vi "Check FET Test.vi"() -> ()   [LabVIEW 2009]
panel:
  in  "STOP":bool
  in  "Check FET":bool
  out "FETs on?":bool=TRUE
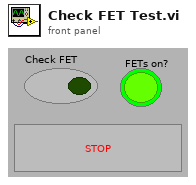
[diagram p1: front panel]
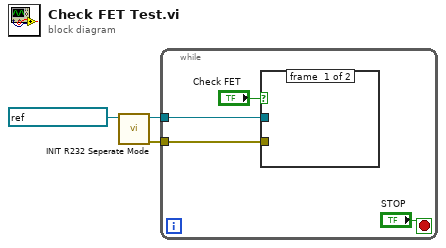
[diagram p0: block diagram]
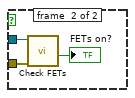
[diagram p2: hidden frame]
diagram:
  n1 = call "INIT R232 Seperate Mode.vi"("MC VISA resource in"=refnum<visa-resource-name> "ASRL1::INSTR") -> ("MC error out"=w1:errorcluster, "MC VISA resource  out"=w2:refnum<visa-resource-name>)  [unwired: 8 in, 1 out]
  n2 = while {
    tunnel: w2 -> [w7]
    tunnel: w1 -> [w6]
    stop <- "STOP" stop-if-true
    n3 = case shown="True" "Check FET" {
      tunnel: w7 -> [_ w10]
      tunnel: w6 -> [_ w9]
      frame #0 {
      }
      frame #1 {
        n4 = call "Check FETs.vi"("error in (no error)"=w9, "MC VISA resource in"=w10) -> ("FETs on?"=→"FETs on?":bool)  [unwired: 5 in, 4 out]
      }
    }
  }
